vi "Read Frequency.vi"(8 "error in":errorcluster, 11 "PWM output channel in":refnum<class "PWM Output Channel.lvclass">) -> (0 "error out":errorcluster, 2 "frequency":T1, 3 "PWM output channel out":refnum<class "PWM Output Channel.lvclass">)   [LabVIEW 2017, in "Scan Engine Scripting.lvlib" / "PWM Output Channel.lvclass"]
uses:
  PWM Output Channel.lvclass
  Frequency.ctl
  PWM Output Channel.lvclass/PWM Output Channel.ctl
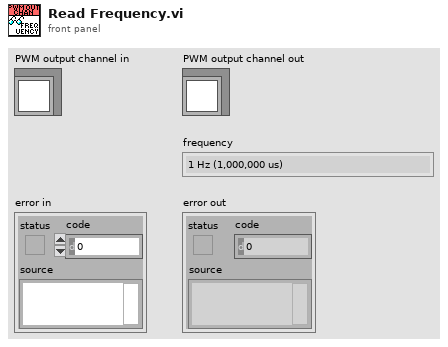
[diagram p1: front panel]
types:
  T1 = typedef "Scan Engine Scripting.lvlib/PWM Output Channel.lvclass/Frequency.ctl" = enum16{"1 Hz (1,000,000 us)", "50 Hz (20,000 us)", "250 Hz (4,000 us)", "500 Hz (2,000 us)", "1 kHz (1,000 us)", "5 kHz (200 us)", "10 kHz (100 us)", "20 kHz (50 us)"}
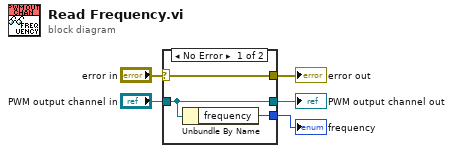
[diagram p0: block diagram]
diagram:
  n1 = case shown="No Error" "error in" {
    selector: "error in" -> [w8 w9]
    tunnel: [w8 w9] -> w4
    tunnel: [w7 w10] -> w2
    tunnel: "PWM output channel in" -> [w7 w10]
    tunnel: [w6 _] -> w1
    frame No Error {
      n2 = Unbundle By Name(w7) -> ("frequency"=w6:T1)
    }
    frame Error {
    }
  }
  "error out" <- w4
  "PWM output channel out" <- w2
  "frequency" <- w1
